vi "Select Sheet.vi"(7 "Sheet (0)":i32, 8 "error in (no error)":errorcluster, 11 "Excel XML in":refnum<class "Excel XML.lvclass">) -> (0 "error out":errorcluster, 3 "Excel XML out":refnum<class "Excel XML.lvclass">)   [LabVIEW 2013, in "Excel XML.lvclass"]
uses:
  Excel XML.lvclass
  Spreadsheet.lvclass
  Excel XML.lvclass/Excel XML.ctl
  C:/PhaeronGit/LVNPOI/Resources/NPOI 2.1.1 dotnet4/NPOI.OOXML.dll
  Resources/NPOI 2.1.1 dotnet4/NPOI.OOXML.dll
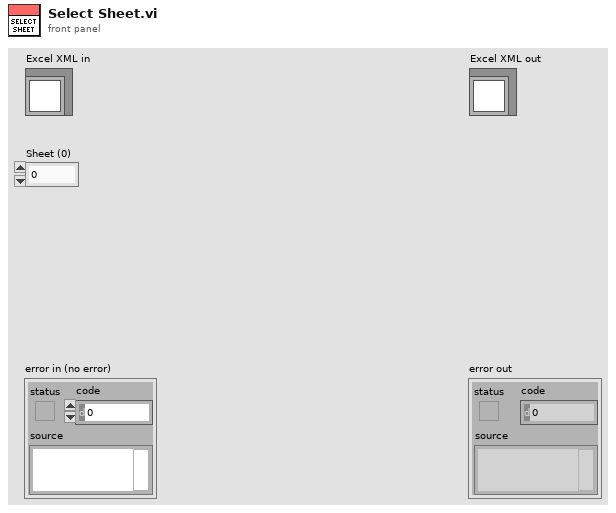
[diagram p1: front panel]
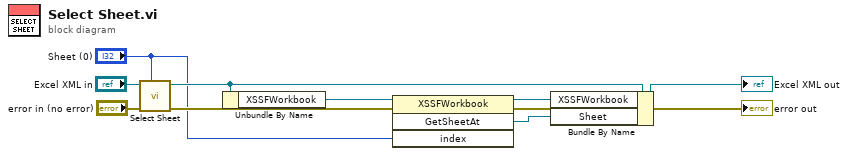
[diagram p0: block diagram]
diagram:
  n1 = call-parent "Select Sheet.vi"("Sheet (0)"="Sheet (0)", "error in (no error)"="error in (no error)", "Spreadsheet in"="Excel XML in") -> ("error out"=w6:errorcluster, "Spreadsheet out"=w2:refnum<class "Excel XML.lvclass">)  [unwired: 7 in]
  n2 = Unbundle By Name(w2) -> ("XSSFWorkbook"=w8:refnum<k24>)
  n3 = invoke class="XSSFWorkbook" method="GetSheetAt"(reference=w8, error in=w6, "index"="Sheet (0)") -> (reference out=w3:refnum<k24>, error out=→"error out":errorcluster, "GetSheetAt"=w7:refnum<k24>)  [unwired: 1 in, 1 out]
  n4 = Bundle By Name(cluster=w2, "XSSFWorkbook"=w3, "Sheet"=w7) -> (→"Excel XML out":refnum<class "Excel XML.lvclass">)
